vi "ALR handlingB.vi"(0 "ALR_State in":T6, 1 "Alarms.ALR_defs":T1, 2 "connect":bool[](array[boolean]), 3 "On":bool=TRUE, 5 "ALR_ON_OFF":T2, 7 "ALRParam":T3, 11 "error in (no error)":errorcluster, 12 "Sensor state":T7[](array[typedef]), 13 "di_sens_state":bool[](array[boolean]), 14 "RESET all":bool) -> (4 "ALR_State":T6, 15 "error out":errorcluster)   [LabVIEW 2019, in "Alarms.lvlib"]
uses:
  Alarms.lvlib
  Inputs/Ctl/Parameter State.ctl
  Ctl/ALRs_State.ctl
  Ctl/ALR_Parameters.ctl
  Ctl/ALR code.ctl
  Ctl/ALR type.ctl
  Ctl/ALR_ON_OFF.ctl
  Ctl/ALR_defs.ctl
  Logik/fronts_ext.vi
  Trigers/RS_ext.vi
  Counter/Counter.lvlib
  Timer Delay/Timers.lvlib
  Trigers/Triggers.lvlib
  Logik/Logik.lvlib
  Inputs/Inputs.lvlib
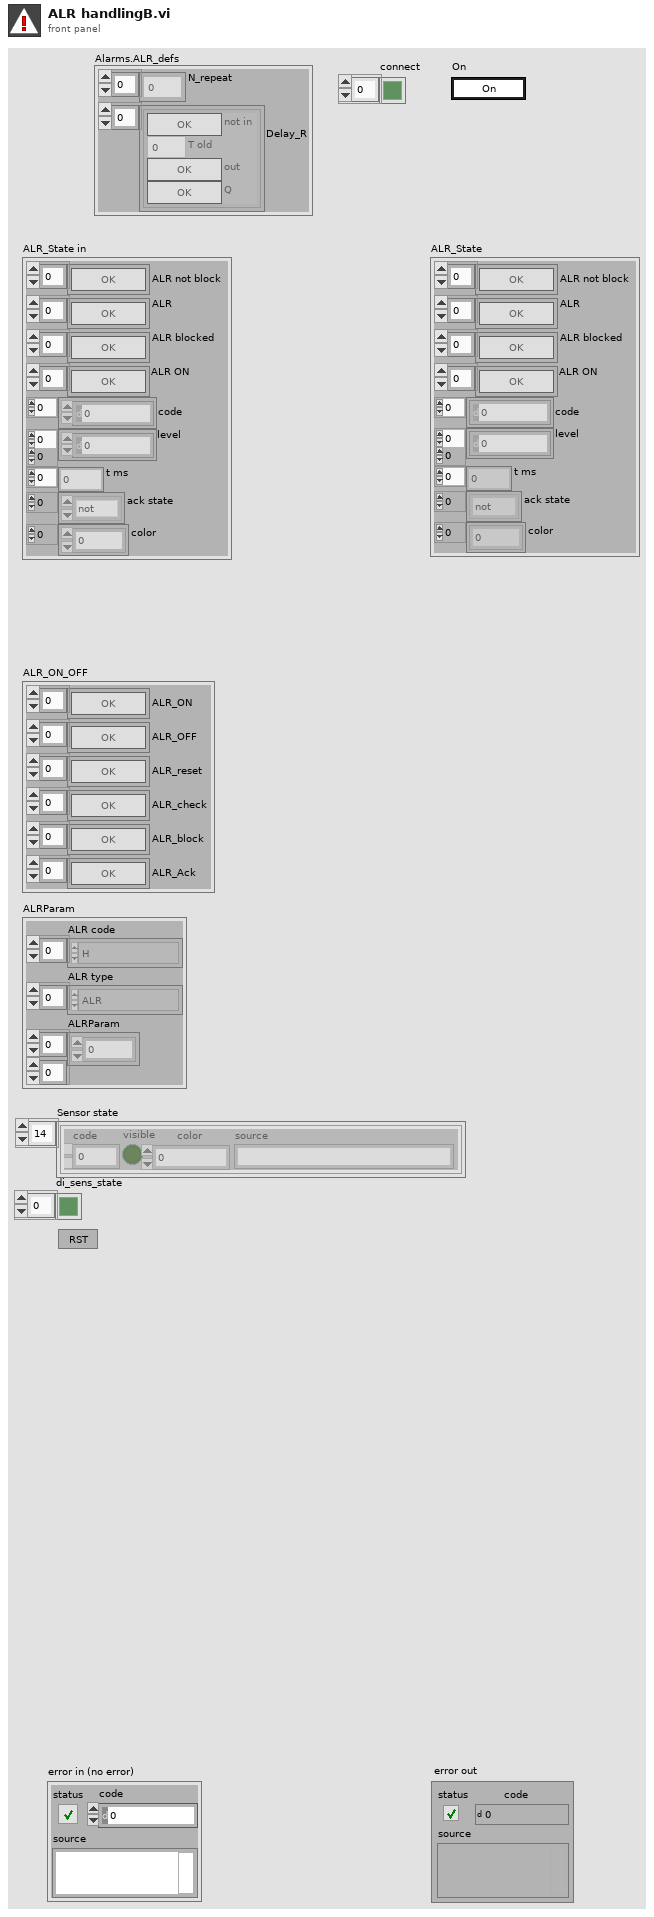
[diagram p1: front panel]
types:
  T1 = typedef "Alarms.lvlib/ALR_defs.ctl" = cluster{"N_repeat":u32[], "Delay_R":cluster{"not in":bool, "T old":u32, "out":bool, "Q":bool}[]}
  T2 = typedef "Alarms.lvlib/ALR_ON_OFF.ctl" = cluster{"ALR_ON":bool[], "ALR_OFF":bool[], "ALR_reset":bool[], "ALR_check":bool[], "ALR_block":bool[], "ALR_Ack":bool[]}
  T3 = typedef "Alarms.lvlib/ALR_Parameters.ctl" = cluster{"ALR code":T4[], "ALR type":T5[], "ALRParam":u32[][]}
  T4 = typedef "Alarms.lvlib/ALR code.ctl" = enum16{"CONN", "H", "HH", "L", "LL", "SERR", "ON", "OFF", "XM19", "XM24", "XM47", "XM51", "XM52", "XM53", "XM54", "XM55", "XM56", "XM61", "XM62", "XM63", "XM64", "XM65", "XM66"}
  T5 = typedef "Alarms.lvlib/ALR type.ctl" = enum16{"ACD", "ACDR", "ALRN", "ALR"}
  T6 = typedef "Alarms.lvlib/ALRs_State.ctl" = cluster{"ALR not block":bool[], "ALR":bool[], "ALR blocked":bool[], "ALR ON":bool[], "code":i32[], "level":i32[][], "t ms":u32[], "ack state":enum32{"not", "tripped", "reset", "ack"}[], "color":u32[]}
  T7 = typedef "Inputs.lvlib/Parameter State.ctl" = cluster{"code":i32, "visible":bool, "color":u32, "source":string}
  T8 = cluster{"not in":bool, "T old":u32, "out":bool, "Q":bool}[]
  T9 = cluster{"not in":bool, "T old":u32, "out":bool, "Q":bool}
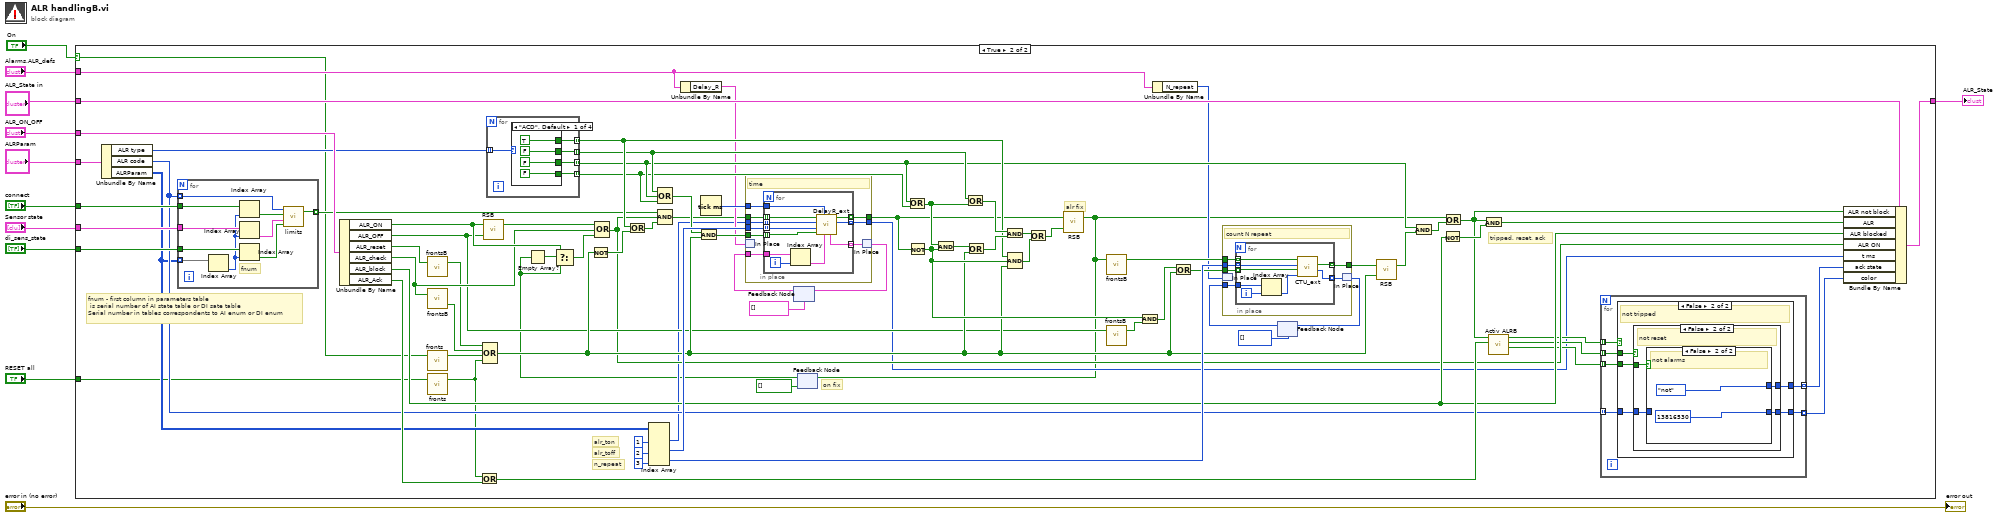
[diagram p0: block diagram]
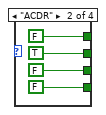
[diagram p3: hidden frame]
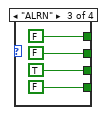
[diagram p4: hidden frame]
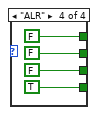
[diagram p5: hidden frame]
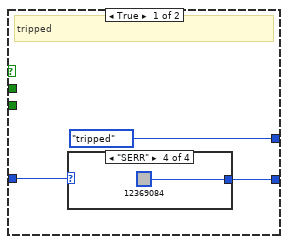
[diagram p6: hidden frame]
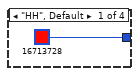
[diagram p7: hidden frame]
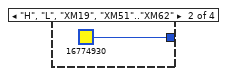
[diagram p8: hidden frame]
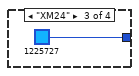
[diagram p9: hidden frame]
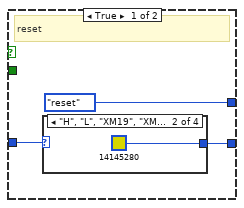
[diagram p10: hidden frame]
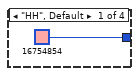
[diagram p11: hidden frame]
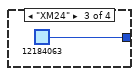
[diagram p12: hidden frame]
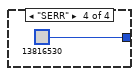
[diagram p13: hidden frame]
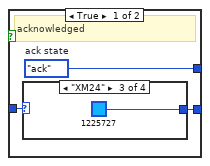
[diagram p14: hidden frame]
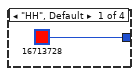
[diagram p15: hidden frame]
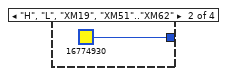
[diagram p16: hidden frame]
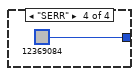
[diagram p17: hidden frame]
diagram:
  n1 = case shown="True" "On" {
    selector: "On" -> [_ w16]
    tunnel: "connect" -> [_ w94]
    tunnel: "Sensor state" -> [_ w93]
    tunnel: "di_sens_state" -> [_ w92]
    tunnel: "RESET all" -> [_ w17]
    tunnel: [w12 w91] -> w7
    tunnel: "ALR_State in" -> [w12 w90]
    tunnel: "ALRParam" -> [_ w89]
    tunnel: "ALR_ON_OFF" -> [_ w88]
    tunnel: "Alarms.ALR_defs" -> [_ w87]
    frame False {
    }
    frame True {
      # "tripped, reset, ack"
      # "alr fix"
      # "n_repeat"
      # "alr_toff"
      # "alr_ton"
      # "on fix"
      # "fnum - first column in parameters table\n is serial number of AI state table or DI sate table\nSerial number in tables correspondents to AI enum or DI enum"
      n2 = Unbundle By Name(w89) -> ("ALR type"=w34:T5[], "ALR code"=w35:T4[], "ALRParam"=w33:u32[][])
      n3 = for {
        tunnel: w33 -> [w116] mode=indexing
        tunnel: w93 -> [w115]
        tunnel: w92 -> [w114]
        tunnel: w35 -> [w113] mode=indexing
        tunnel: w94 -> [w111]
        tunnel: [w109] -> w36 mode=indexing
        # "fnum"
        n4 = Index Array(array=w116) -> (element=w110:u32)  [unwired: 1 in]
        n5 = Index Array(array=w111, index=w110) -> (element=w112:bool)
        n6 = Index Array(array=w115, index=w110) -> (element=w118:T7)
        n7 = Index Array(array=w114, index=w110) -> (element=w117:bool)
        n8 = call "limits.vi"("ON"=w117, "STATE"=w118, "CONN"=w112, "ALR code"=w113) -> ("LIMIT"=w109:bool)  [unwired: 1 in]
      }
      n9 = Unbundle By Name(w88) -> ("ALR_ON"=w53:bool[], "ALR_OFF"=w45:bool[], "ALR_reset"=w48:bool[], "ALR_check"=w52:bool[], "ALR_block"=w43:bool[], "ALR_Ack"=w50:bool[])
      n10 = call "frontsB.vi"("IN"=w48) -> ("RAISE"=w47:bool[])  [unwired: 1 in, 1 out]
      n11 = call "frontsB.vi"("IN"=w52) -> ("FALL"=w46:bool[])  [unwired: 1 in, 1 out]
      n12 = call "fronts.vi"("in"=w16) -> ("raise"=w14:bool)  [unwired: 1 in, 1 out]
      n13 = call "fronts.vi"("in"=w17) -> ("raise"=w15:bool)  [unwired: 1 in, 1 out]
      n14 = Or(x=w15, y=w50) -> (x .or. y?=w51:bool[])
      n15 = Compound Arithmetic op=OR(w47, w46, w14, w15) -> (w66:bool[])
      n16 = call "RSB.vi"("R"=w45, "S"=w53) -> ("Q"=w85:bool[])  [unwired: 1 out]
      n17 = for {
        tunnel: w34 -> [w123] mode=indexing
        tunnel: [w122] -> w64 mode=indexing
        tunnel: [w121] -> w63 mode=indexing
        tunnel: [w120] -> w62 mode=indexing
        tunnel: [w119] -> w61 mode=indexing
        n18 = case shown="\"ACD\", Default" w123 {
          tunnel: [TRUE FALSE FALSE FALSE] -> w122
          tunnel: [FALSE TRUE FALSE FALSE] -> w121
          tunnel: [FALSE FALSE TRUE FALSE] -> w120
          tunnel: [FALSE FALSE FALSE TRUE] -> w119
          frame "ACD", Default {
          }
          frame "ACDR" {
          }
          frame "ALRN" {
          }
          frame "ALR" {
          }
        }
      }
      n19 = Not(x=w66) -> (.not. x?=w82:bool[])
      n20 = Or(x=w64, y=w82) -> (x .or. y?=w83:bool[])
      n21 = Index Array(array=w33, index (col) #1=1 ("disabled index (col)"), index (col) #2=2 ("disabled index (col)"), index (col) #3=3 ("disabled index (col)")) -> (element #1=w26:u32[], element #2=w70:u32[], element #3=w69:u32[])  [unwired: 3 in]
      n22 = Compound Arithmetic op=OR(w63, w62, w61) -> (w65:bool[])
      n23 = Unbundle By Name(w87) -> ("Delay_R"=w32:T8)
      n24 = And(x=w65, y=w66) -> (x .and. y?=w57:bool[])
      n25 = Tick Count (ms)() -> (millisecond timer value=w49:u32)
      n26 = feedback #1(T8 [] ("Delay_R")) -> (w30:T8)
      n27 = feedback #2(bool[] [] ("Q")) -> (w21:bool[])
      n28 = Empty Array?(array=w21) -> (empty?=w54:bool)
      n29 = Select(t=w53, s=w54, f=w21) -> (s? t:f=w55:bool[])
      n30 = Compound Arithmetic op=OR(w85, w52, w55) -> (w42:bool[])
      n31 = Compound Arithmetic op=AND(w36, w42, w83) -> (w28:bool[])
      n32 = in-place {
        in-place-border: w70 -> [w148]
        in-place-border: w57 -> [w147]
        in-place-border: w49 -> [w146]
        in-place-border: w30 -> [w144]
        in-place-border: [w143] -> w29
        in-place-border: w28 -> [w142]
        in-place-border: [w141] -> w27
        in-place-border: w26 -> [w140]
        # "time"
        n33 = in-place-match #3(w32) -> ()  [unwired: 1 out]
        n34 = for {
          tunnel: w140 -> [w159] mode=indexing
          tunnel: w148 -> [w158] mode=indexing
          tunnel: [w157] -> w141 mode=indexing
          tunnel: [w156] -> w143 mode=indexing
          tunnel: w147 -> [w155] mode=indexing
          tunnel: w142 -> [w154] mode=indexing
          tunnel: [w153] -> w145 mode=indexing
          tunnel: w146 -> [w152]
          tunnel: w144 -> [w150]
          i -> [w151]
          n35 = Index Array(array=w150, index=w151) -> (element=w149:T9)
          n36 = call "DelayR_ext.vi"("DelayR reg old"=w149, "T  ms (0 curr)"=w152, "R"=w155, "DelayOff (0)"=w158, "DelayOn (0)"=w159, "In"=w154) -> ("t ms"=w157:u32, "Out"=w156:bool, "DelayR reg"=w153:T9)  [unwired: 3 in]
        }
        n37 = in-place-match #3(w145) -> (w31:T8)
      }
      n38 = feedback-in #1(w31) -> ()
      n39 = Or(x=w62, y=w61) -> (x .or. y?=w68:bool[])
      n40 = Not(x=w29) -> (.not. x?=w76:bool[])
      n41 = And(x=w68, y=w76) -> (x .and. y?=w84:bool[])
      n42 = Or(x=w63, y=w68) -> (x .or. y?=w67:bool[])
      n43 = Or(x=w84, y=w66) -> (x .or. y?=w80:bool[])
      n44 = And(x=w67, y=w80) -> (x .and. y?=w79:bool[])
      n45 = Compound Arithmetic op=AND(w64, w76, w66) -> (w78:bool[])
      n46 = Or(x=w79, y=w78) -> (x .or. y?=w81:bool[])
      n47 = call "RSB.vi"("R"=w81, "S"=w29) -> ("Q"=w22:bool[])  [unwired: 1 out]
      n48 = feedback-in #2(w22) -> ()
      n49 = call "frontsB.vi"("IN"=w22) -> ("RAISE"=w60:bool[])  [unwired: 1 in, 1 out]
      n50 = call "frontsB.vi"("IN"=w45) -> ("RAISE"=w75:bool[])  [unwired: 1 in, 1 out]
      n51 = And(x=w76, y=w75) -> (x .and. y?=w77:bool[])
      n52 = Unbundle By Name(w87) -> ("N_repeat"=w25:u32[])
      n53 = Or(x=w77, y=w66) -> (x .or. y?=w59:bool[])
      n54 = feedback #4(u32[] [] ("N_repeat")) -> (w23:u32[])
      n55 = in-place {
        in-place-border: w69 -> [w100]
        in-place-border: w60 -> [w99]
        in-place-border: w59 -> [w98]
        in-place-border: [w97] -> w58
        in-place-border: w23 -> [w96]
        # "count N repeat"
        n56 = in-place-match #5(w25) -> ()  [unwired: 1 out]
        n57 = for {
          tunnel: [w108] -> w97 mode=indexing
          tunnel: w98 -> [w107] mode=indexing
          tunnel: w99 -> [w106] mode=indexing
          tunnel: [w105] -> w95 mode=indexing
          tunnel: w100 -> [w104] mode=indexing
          tunnel: w96 -> [w103]
          i -> [w102]
          n58 = Index Array(array=w103, index=w102) -> (element=w101:u32)
          n59 = call "CTU_ext.vi"("DO old"=w101, "R"=w107, "DI"=w104, "IN"=w106) -> ("DO"=w105:u32, "EU"=w108:bool)  [unwired: 2 in]
        }
        n60 = in-place-match #5(w95) -> (w24:u32[])
      }
      n61 = feedback-in #4(w24) -> ()
      n62 = call "RSB.vi"("R"=w66, "S"=w58) -> ("Q"=w56:bool[])  [unwired: 1 out]
      n63 = And(x=w62, y=w56) -> (x .and. y?=w74:bool[])
      n64 = Not(x=w43) -> (.not. x?=w86:bool[])
      n65 = Or(x=w22, y=w74) -> (x .or. y?=w13:bool[])
      n66 = And(x=w13, y=w86) -> (x .and. y?=w44:bool[])
      n67 = call "Activ ALRB.vi"("Ack"=w51, "ALR"=w13) -> ("A alr"=w41:bool[], "R alr"=w40:bool[], "T alr"=w39:bool[])  [unwired: 7 in]
      n68 = for {
        tunnel: w40 -> [w165] mode=indexing
        tunnel: w41 -> [w164] mode=indexing
        tunnel: w39 -> [w160] mode=indexing
        tunnel: w35 -> [w163] mode=indexing
        tunnel: [w162] -> w38 mode=indexing
        tunnel: [w161] -> w37 mode=indexing
        n69 = case shown="False" w160 {
          tunnel: [enum32{"not", "tripped", "reset", "ack"}."tripped" ("X3(MenuSetSate)") w177] -> w162
          tunnel: w165 -> [_ w173]
          tunnel: w164 -> [_ w176]
          tunnel: w163 -> [w166 w175]
          tunnel: [w167 w174] -> w161
          frame True {
            # "tripped"
            n70 = case shown="\"SERR\"" w166 {
              tunnel: [u32 16713728 ("Color Box") u32 16774930 ("Color Box") u32 1225727 ("Color Box") u32 12369084 ("Color Box 2")] -> w167
              frame "HH", Default {
              }
              frame "H", "L", "XM19", "XM51".."XM62" {
              }
              frame "XM24" {
              }
              frame "SERR" {
              }
            }
          }
          frame False {
            # "not tripped"
            n71 = case shown="False" w173 {
              tunnel: [enum32{"not", "tripped", "reset", "ack"}."reset" ("X3(MenuSetSate)") w188] -> w177
              tunnel: w176 -> [_ w185]
              tunnel: w175 -> [w178 w187]
              tunnel: [w179 w186] -> w174
              frame True {
                # "reset"
                n72 = case shown="\"H\", \"L\", \"XM19\", \"XM51\"..\"XM62\"" w178 {
                  tunnel: [u32 16754854 ("Color Box") u32 14145280 ("Color Box 2") u32 12184063 ("Color Box 2") u32 13816530 ("Color Box 2")] -> w179
                  frame "HH", Default {
                  }
                  frame "H", "L", "XM19", "XM51".."XM62" {
                  }
                  frame "XM24" {
                  }
                  frame "SERR" {
                  }
                }
              }
              frame False {
                # "not reset"
                n73 = case shown="False" w185 {
                  tunnel: [w191 enum32{"not", "tripped", "reset", "ack"}."not" ("X3(MenuSetSate)")] -> w188
                  tunnel: w187 -> [w190 _]
                  tunnel: [w189 u32 13816530 ("color")] -> w186
                  frame True {
                    w191 = enum32{"not", "tripped", "reset", "ack"}."ack"  # ack state
                    # "acknowledged"
                    n74 = case shown="\"XM24\"" w190 {
                      tunnel: [u32 16713728 ("Color Box") u32 16774930 ("Color Box") u32 1225727 ("Color Box") u32 12369084 ("Color Box 2")] -> w189
                      frame "HH", Default {
                      }
                      frame "H", "L", "XM19", "XM51".."XM62" {
                      }
                      frame "XM24" {
                      }
                      frame "SERR" {
                      }
                    }
                  }
                  frame False {
                    # "not alarms"
                  }
                }
              }
            }
          }
        }
      }
      n75 = Bundle By Name(cluster=w90, "ALR not block"=w13, "ALR"=w44, "ALR blocked"=w43, "ALR ON"=w42, "t ms"=w27, "ack state"=w38, "color"=w37) -> (w91:T6)
    }
  }
  "ALR_State" <- w7
  "error out" <- "error in (no error)"
